vi "Vision Processing.vi"(4 "error in (no error)":errorcluster, 5 "Camera Type":enum16{"206", "1011"}(ring), 6 "Camera Name":string="Camera") -> ()   [LabVIEW 2013]
uses:
  Robot Global Data.vi
  <vilib>/vision/NI_Vision_Development_Module.lvlib
panel:
  in  "View":bool
  out "Target Info":T1(array[cluster])=[{"Center Position"={"X"=20.549999999999997, "Y"=12.8}, "Distance (ft)"=10.081642317668745, "Center"=TRUE}]
  in  "Area Size Limit %":dbl=0.5
  in  "Particle Count Limit":i32=8
  in  "Score Limits":T2={"Rect Coverage"=60.0, "X Edge Strength"=40.0, "Y Edge Strength"=60.0, "Center"=75.0, "Outer"=75.0}
  in  "Processing":enum32{"Color", "Monochrome"}(tab)
  out "Value":cluster{i32, i32}={246, 255}
  out "Saturation":cluster{i32, i32}={246, 255}
  out "Hue":cluster{i32, i32}={94, 160}
  in  "Luminance":i32=255
  in  "Saturation":i32=255
  in  "Hue":i32(knob)=127 scale=0.0..255.0
  in  "Margins":cluster{"Hue":i32, "Sat":i32, "Val":i32}={"Hue"=80, "Sat"=80, "Val"=80} {"Sat" scale=0.0..80.0; "Val" scale=0.0..80.0; "Hue" scale=0.0..80.0}
  in  "Range":cluster{"Lower value":sgl, "Upper value":sgl}={"Lower value"=150.0, "Upper value"=255.0} {"Lower value" scale=0.0..255.0; "Upper value" scale=0.0..255.0}
  in  "View":bool
  out "Processed Image":T3(plugin-control)
  out "Original Image":T3(plugin-control)
  # "Instructions:\nProcessing the reflective tape that is illuminated by a ring light can be based\non color or light intensity.\nParticles within the image are scored by rectangle coverage, aspect ratio, and\nfor being hollow with a bold edge. A particle is considered a target if all scores\nare above the score limits. Particles can be annotated -- surrounded by\na rectangle and scores drawn to the left .\nTo control the number of particles being scored, use the count limit and the size\nlimit."
  # "To debug, Enable using the View button.\nFor color processing, you can click in the image to select the color for processing."
  # "Enable by clicking the View button.\nGreen scores are above the limit, orange are below. Inner/outer rect\nindicates all passed."
  # "Lower/Upper"
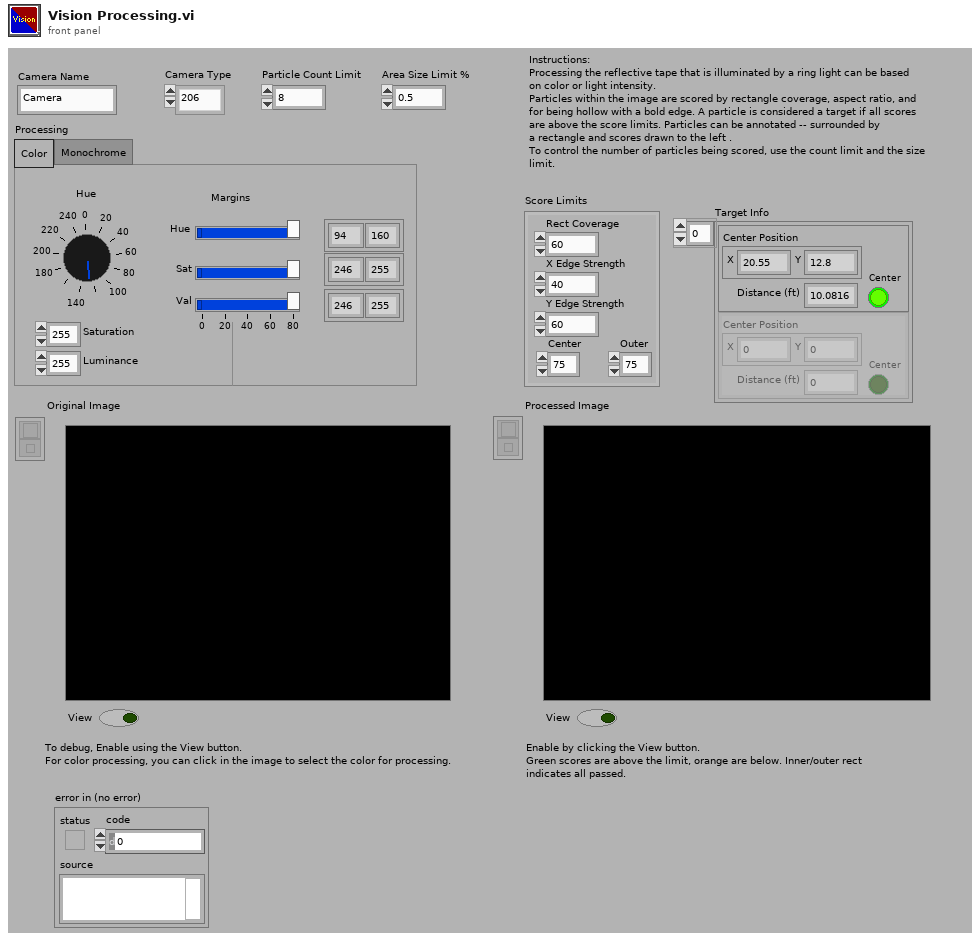
[diagram p1: front panel]
types:
  T1 = cluster{"Center Position":cluster{"X":dbl, "Y":dbl}, "Distance (ft)":dbl, "Center":bool}[]
  T2 = cluster{"Rect Coverage":dbl, "X Edge Strength":dbl, "Y Edge Strength":dbl, "Center":dbl, "Outer":dbl}
  T3 = typedef "IMAQ Image.ctl" = refnum<image>
  T4 = typedef "Image Type" = u32
  T5 = typedef "WPI_CameraDevRef.ctl" = cluster{"Camera Address":string, "CameraStatus":errorcluster, "Acquire Image Notifier":refnum<notifier>}
  T6 = cluster{"Position":cluster{"X":dbl, "Y":dbl}, "Distance (ft)":dbl, "Center":bool}[]
  T7 = typedef "WPI_CameraImageSize.ctl" = enum16{"640x480", "320x240", "160x120"}
  T8 = cluster{cluster{"Left":dbl, "Top":dbl, "Right":dbl, "Bottom":dbl}, "Scores":dbl[], cluster{"Long":dbl, "Short":dbl}}[]
  T9 = cluster{"Target Angles":cluster{"X":dbl, "Y":dbl}, "Distance (ft)":dbl, "Center Target":bool}
  T10 = cluster{"Target Angles":cluster{"X":dbl, "Y":dbl}, "Distance (ft)":dbl, "Center Target":bool}[]
  T11 = cluster{"Left":dbl, "Top":dbl, "Right":dbl, "Bottom":dbl}
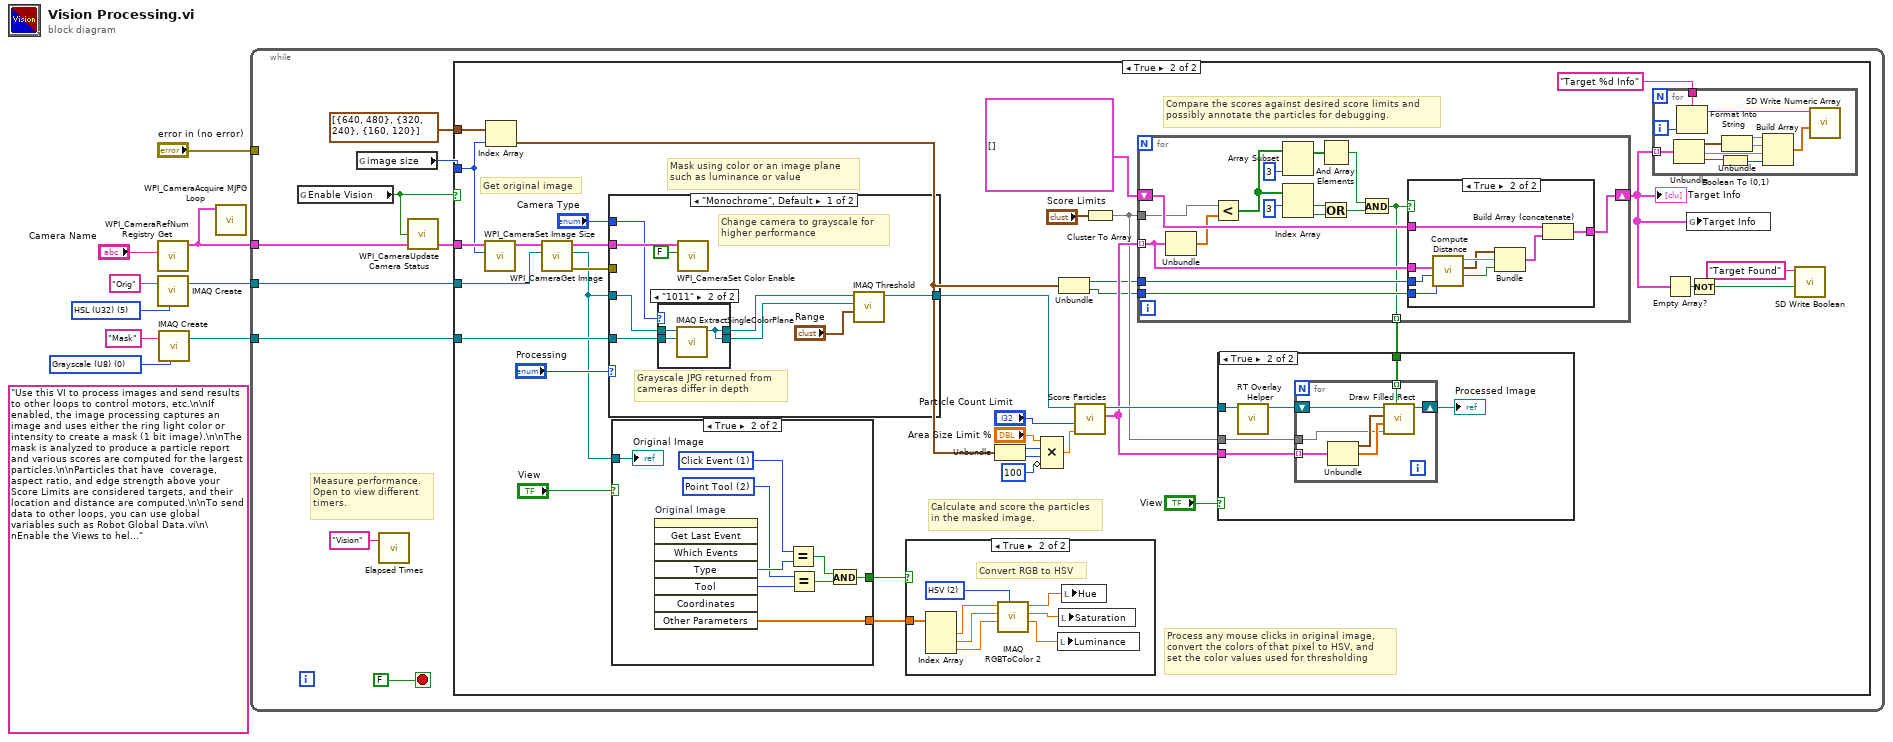
[diagram p0: block diagram]
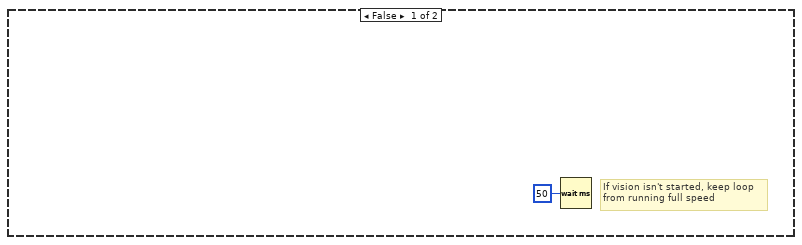
[diagram p2: hidden frame]
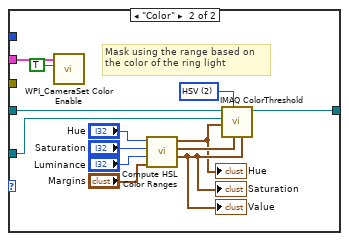
[diagram p5: hidden frame]
diagram:
  w3 = T4 0 items=["Grayscale (U8)", "Grayscale (I16)", "Grayscale (SGL)", "Complex (CSG)", "RGB (U32)", "HSL (U32)", "RGB (U64)", "Grayscale (U16)"] ("Image Type")
  (unwired) "Use this VI to process images and send results to other loops to control motors, etc.\n\nIf enabled, the image processing captures an image and uses either the ring light color or intensity to create a mask (1 bit image).\n\nThe mask is analyzed to produce a particle report and various scores are computed for the largest particles.\n\nParticles that have  coverage, aspect ratio, and edge strength above your Score Limits are considered targets, and their location and distance are computed.\n\nTo send data to other loops, you can use global variables such as Robot Global Data.vi\n\nEnable the Views to help debug color settings. Disable the View to speed up processing."
  w8 = T4 5 items=["Grayscale (U8)", "Grayscale (I16)", "Grayscale (SGL)", "Complex (CSG)", "RGB (U32)", "HSL (U32)", "RGB (U64)", "Grayscale (U16)"] ("Image Type")
  n1 = call <vilib>:"WPI_CameraRefNum Registry Get.vi"("refnum name"="Camera Name") -> ("CameraDevRef"=w5:T5)  [unwired: 9 in, 1 out]
  n2 = call "IMAQ Create"("Image Name"="Orig", "Image Type"=w8) -> ("New Image"=w7:T3)  [unwired: 2 in, 2 out]
  n3 = call "IMAQ Create"("Image Name"="Mask", "Image Type"=w3) -> ("New Image"=w1:T3)  [unwired: 2 in, 2 out]
  n4 = call <vilib>:"WPI_CameraAcquire MJPG Loop.vi"("CameraDevRef"=w5) -> ()  [unwired: 11 in]
  n5 = while {
    tunnel: w7 -> [w17]
    tunnel: w5 -> [w16]
    tunnel: "error in (no error)" -> [_]
    tunnel: w1 -> [w12]
    stop <- FALSE stop-if-true
    # "Measure performance.\nOpen to view different\ntimers."
    n6 = global read "Robot Global Data.vi" "Enable Vision"() -> (w10:bool)
    n7 = global read "Robot Global Data.vi" "image size"() -> (w13:T7)
    n8 = call "Elapsed Times.vi"("Call Name"="Vision") -> ()  [unwired: 2 in, 1 out]
    n9 = call <vilib>:"WPI_CameraUpdate Camera Status.vi"("CameraDevRef In"=w16, "Enable Vision"=w10) -> ("CameraDevRef Out"=w15:T5)  [unwired: 3 in]
    n10 = case shown="True" w10 {
      tunnel: w17 -> [_ w48]
      tunnel: w15 -> [_ w44]
      tunnel: w13 -> [_ w39]
      tunnel: w12 -> [_ w35]
      tunnel: cluster{i32, i32}[] [{640, 480}, {320, 240}, {160, 120}] -> [_ w38]
      frame False {
        # "If vision isn't started, keep loop\nfrom running full speed"
        n11 = Wait (ms)(milliseconds to wait=u32 50) -> ()  [unwired: 1 out]
      }
      frame True {
        # "Compare the scores against desired score limits and\npossibly annotate the particles for debugging."
        # "Process any mouse clicks in original image,\nconvert the colors of that pixel to HSV, and\nset the color values used for thresholding"
        # "Calculate and score the particles\nin the masked image."
        # "Mask using color or an image plane\nsuch as luminance or value"
        # "Get original image"
        n12 = call <vilib>:"WPI_CameraSet Image Size.vi"("Image Size"=w39, "CameraDevRef"=w44) -> ("CameraDevRef Out"=w45:T5)  [unwired: 8 in, 1 out]
        n13 = Index Array(array=w38, index=w39) -> (element=w24:cluster{i32, i32})
        n14 = call <vilib>:"WPI_CameraGet Image.vi"("Image"=w48, "CameraDevRef"=w45) -> ("error out"=w46:errorcluster, "Image Out"=w34:T3, "CameraDevRef Out"=w47:T5)  [unwired: 7 in]
        n15 = case shown="\"Monochrome\", Default" "Processing" {
          tunnel: w34 -> [w79 w101]
          tunnel: [w82 w100] -> w42
          tunnel: w47 -> [w80 w93]
          tunnel: w46 -> [_ _]
          tunnel: w35 -> [w78 w91]
          tunnel: "Camera Type" -> [w77 _]
          frame "Monochrome", Default {
            # "Grayscale JPG returned from\ncameras differ in depth"
            # "Change camera to grayscale for\nhigher performance"
            n16 = case shown="\"1011\"" w77 {
              tunnel: w79 -> [w85 w88]
              tunnel: w78 -> [w84 w87]
              tunnel: [w85 w86] -> w76
              tunnel: [w84 w86] -> w75
              frame "206", Default {
              }
              frame "1011" {
                n17 = call "IMAQ ExtractSingleColorPlane"("Image Dst"=w87, "Image Src"=w88) -> ("Image Dst Out"=w86:T3)  [unwired: 8 in, 1 out]
              }
            }
            n18 = call <vilib>:"WPI_CameraSet Color Enable.vi"("Color Enabled"=FALSE, "CameraDevRef"=w80) -> ()  [unwired: 8 in, 2 out]
            n19 = call "IMAQ Threshold"("Range"="Range", "Image Dst"=w75, "Image Src"=w76) -> ("Image Dst Out"=w82:T3)  [unwired: 3 in, 5 out]
          }
          frame "Color" {
            w99 = u16 2 items=["RGB", "HSL", "HSV", "HSI"] ("Color Mode")
            # "Mask using the range based on\nthe color of the ring light"
            n20 = call <vilib>:"WPI_CameraSet Color Enable.vi"("Color Enabled"=TRUE, "CameraDevRef"=w93) -> ()  [unwired: 8 in, 2 out]
            n21 = call "Compute HSL Color Ranges.vi"("Margins"="Margins", "Luminance"="Luminance", "Saturation"="Saturation", "Hue"="Hue") -> ("Lum Range"=w90:cluster{i32, i32}, "Sat Range"=w98:cluster{i32, i32}, "Hue Range"=w89:cluster{i32, i32})  [unwired: 5 in]
            "Hue" <- w89
            "Saturation" <- w90
            "Value" <- w90
            n22 = call "IMAQ ColorThreshold"("Blue or Luma or Val or Inten Range"=w90, "Green or Sat Range"=w98, "Color Mode"=w99, "Red or Hue Range"=w89, "Image Dst"=w91, "Image Src"=w101) -> ("Image Dst Out"=w100:T3)  [unwired: 4 in, 1 out]
          }
        }
        n23 = case shown="True" "View" {
          tunnel: w34 -> [_ w123]
          tunnel: [_ w118] -> w41
          tunnel: [_ w115] -> w40
          frame False {
          }
          frame True {
            w116 = 2 items=["None", "Selection Tool", "Point Tool", "Line Tool", "Rectangle Tool", "Oval Tool", "Polygon Tool", "ClosedFreehandTool", "Annulus Tool", "Rotated Rectangle Tool", "Zoom Tool", "Pan Tool", "Polyline Tool", "Freehand Tool"] ("Tool")
            w117 = 1 items=["No Event"=0, "Click Event"=1, "Draw Event"=2, "Size Event"=4, "Scroll Event"=5, "Double Click Event"=8] ("Type")
            n24 = invoke on="Original Image" class="ImageControl" method="Get Last Event"() -> ("Type"=w119:i32, "Tool"=w122:i32, "Other Parameters"=w115:sgl[])  [unwired: 8 in, 5 out]
            n25 = Equal?(x=w117, y=w119) -> (x = y?=w120:bool)
            n26 = Equal?(x=w116, y=w122) -> (x = y?=w121:bool)
            n27 = And(x=w120, y=w121) -> (x .and. y?=w118:bool)
            "Original Image" <- w123
          }
        }
        n28 = case shown="True" w41 {
          tunnel: w40 -> [_ w74]
          frame False {
          }
          frame True {
            w73 = u16 2 items=["RGB", "HSL", "HSV", "HSI", "CIE L*a*b*", "CIE XYZ"] ("Color Mode")
            # "Convert RGB to HSV"
            n29 = Index Array(array=w74) -> (element #1=w72:sgl, element #2=w70:sgl, element #3=w68:sgl)  [unwired: 3 in]
            n30 = call "IMAQ RGBToColor 2"("Color Mode"=w73, "Blue value"=w68, "Green value"=w70, "Red value"=w72) -> ("Blue or Luma or Val or Inten or Z or b*value"=w67:dbl, "Green or Sat or Y or a* value"=w69:dbl, "Red or Hue or X or L* value"=w71:dbl)  [unwired: 4 in, 1 out]
            n31 = local write "Luminance"(w67) -> ()
            n32 = local write "Saturation"(w69) -> ()
            n33 = local write "Hue"(w71) -> ()
          }
        }
        n34 = Unbundle(w24) -> (w28:i32, w27:i32)
        n35 = Compound Arithmetic op=MULTIPLY("Area Size Limit %", w28, w27, invert 100 ("length")) -> (w25:dbl)
        n36 = Unbundle(w24) -> (w37:i32, w36:i32)
        n37 = call "Score Particles.vi"("Area Size Limit"=w25, "Particle Count Limit"="Particle Count Limit", "Image Refnum in"=w42) -> ("Scored Particle Info"=w52:T8, "Image Refnum out"=w54:T3)  [unwired: 7 in]
        n38 = Cluster To Array(cluster="Score Limits") -> (array=w50:dbl[])
        n39 = for {
          shift-right: [w138] -> w22
          shift-left: T6 [] -> [w139]
          tunnel: w37 -> [w137]
          tunnel: w52 -> [w133] mode=indexing
          tunnel: w50 -> [w135]
          tunnel: w36 -> [w134]
          tunnel: [w124] -> w30 mode=indexing
          n40 = Unbundle(w133) -> ("Scores"=w136:dbl[])  [unwired: 2 out]
          n41 = Less?(x=w135, y=w136) -> (x < y?=w125:bool[])
          n42 = Array Subset(array=w125, length=3) -> (w127:bool[])  [unwired: 1 in]
          n43 = Index Array(array=w125, index #1=3 ("length")) -> (element #1=w129:bool, element #2=w130:bool)  [unwired: 1 in]
          n44 = And Array Elements(Boolean array=w127) -> (logical AND=w132:bool)
          n45 = Or(x=w129, y=w130) -> (x .or. y?=w131:bool)
          n46 = And(x=w132, y=w131) -> (x .and. y?=w124:bool)
          n47 = case shown="True" w124 {
            tunnel: w139 -> [w140 w149]
            tunnel: [w140 w148] -> w138
            tunnel: w137 -> [_ w146]
            tunnel: w134 -> [_ w144]
            tunnel: w133 -> [_ w142]
            frame False {
            }
            frame True {
              n48 = call "Compute Distance.vi"("Y Image Resolution"=w144, "X Image Resolution"=w146, "Particle Scores"=w142) -> ("Center Target"=w141:bool, "Target Angles"=w143:cluster{"X":dbl, "Y":dbl}, "Distance (ft)"=w145:dbl)  [unwired: 6 in]
              n49 = Bundle("Target Angles"=w143, "Distance (ft)"=w145, "Center Target"=w141) -> (w147:T9)  [unwired: 1 in]
              n50 = Build Array (concatenate)(w149, w147) -> (w148:T10)
            }
          }
        }
        "Target Info" <- w22
        n51 = case shown="True" "View" {
          tunnel: w54 -> [_ w104]
          tunnel: w52 -> [_ w106]
          tunnel: w50 -> [_ w105]
          tunnel: w30 -> [_ w102]
          frame False {
          }
          frame True {
            n52 = call "RT Overlay Helper.vi"("Refnum in"=w104) -> ("Refnum out"=w107:T3)  [unwired: 10 in]
            n53 = for {
              shift-right: [w113] -> w103
              shift-left: w107 -> [w114]
              tunnel: w106 -> [w110] mode=indexing
              tunnel: w105 -> [w109]
              tunnel: w102 -> [w108] mode=indexing
              n54 = Unbundle(w110) -> (w111:T11, "Scores"=w112:dbl[])  [unwired: 1 out]
              n55 = call "Draw Filled Rect.vi"("Limit Passed"=w108, "Limits"=w109, "Scores"=w112, "Bounding Box"=w111, "image in"=w114) -> ("image out"=w113:T3)  [unwired: 6 in]
            }
            "Processed Image" <- w103
          }
        }
        n56 = for {
          tunnel: w22 -> [w66] mode=indexing
          tunnel: "Target %d Info" ("Name") -> [w65]
          i -> [w62]
          n57 = Unbundle(w66) -> ("Position"=w63:cluster{"X":dbl, "Y":dbl}, "Distance (ft)"=w58:dbl, "Center"=w61:bool)
          n58 = Format Into String(format string=w65, w62) -> (resulting string=w64:string)  [unwired: 2 in, 1 out]
          n59 = Boolean To (0,1)(Boolean=w61) -> (0, 1=w57:i16)
          n60 = Unbundle(w63) -> ("X"=w60:dbl, "Y"=w59:dbl)
          n61 = Build Array(w60, w59, w58, w57) -> (w56:dbl[])
          n62 = call <vilib>:"SD Write Numeric Array.vi"("Numeric Array"=w56, "Name"=w64) -> ()  [unwired: 8 in, 2 out]
        }
        n63 = Empty Array?(array=w22) -> (empty?=w21:bool)
        n64 = global write "Robot Global Data.vi" "Target Info"(w22) -> ()
        n65 = Not(x=w21) -> (.not. x?=w20:bool)
        n66 = call <vilib>:"SD Write Boolean.vi"("Boolean"=w20, "Name"="Target Found") -> ()  [unwired: 8 in, 2 out]
      }
    }
  }
